vi "读取秘钥.vi"(8 "error in (no error)":errorcluster caption="错误输入（无错误）") -> (0 "error out":errorcluster caption="错误输出", 2 "值":string[](array[string]), 3 "包含启动项":bool)   [LabVIEW 2016]
uses:
  <vilib>/registry/registry.llb/Registry RtKey.ctl
  <vilib>/registry/registry.llb/Read Registry Value Simple STR.vi
panel:
  out "名称":string[](array[string])
  in  "簇":cluster{"password":string}={"password"="平台数据发送系统"}
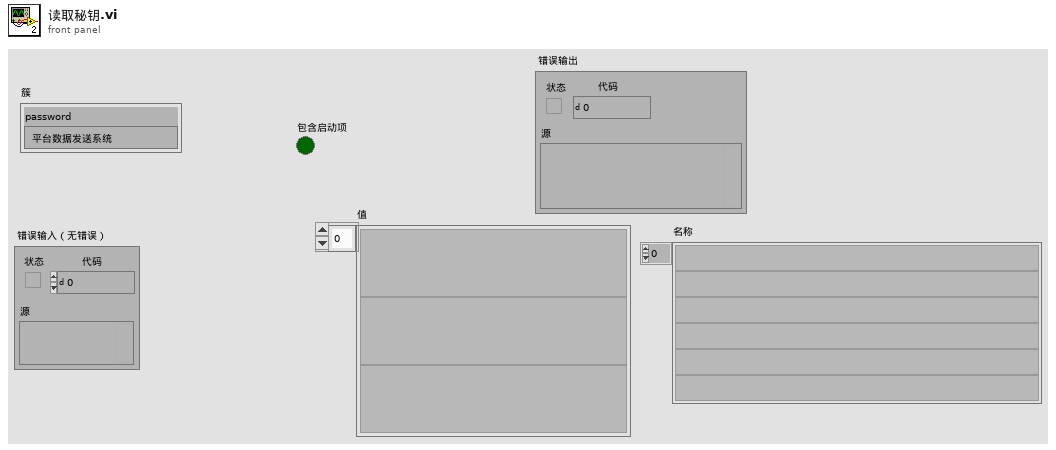
[diagram p1: front panel]
types:
  T1 = typedef "Registry RtKey.ctl" = enum32{"HKEY_CLASSES_ROOT", "HKEY_CURRENT_USER", "HKEY_LOCAL_MACHINE", "HKEY_USERS", "HKEY_PERFORMANCE_DATA", "HKEY_CURRENT_CONFIG", "HKEY_DYN_DATA"}
  T2 = typedef "Registry refnum.ctl" = refnum<k1>
  T3 = cluster{"numValues":i32, "maxValueNameLen":i32, "maxValueDataLen":i32}
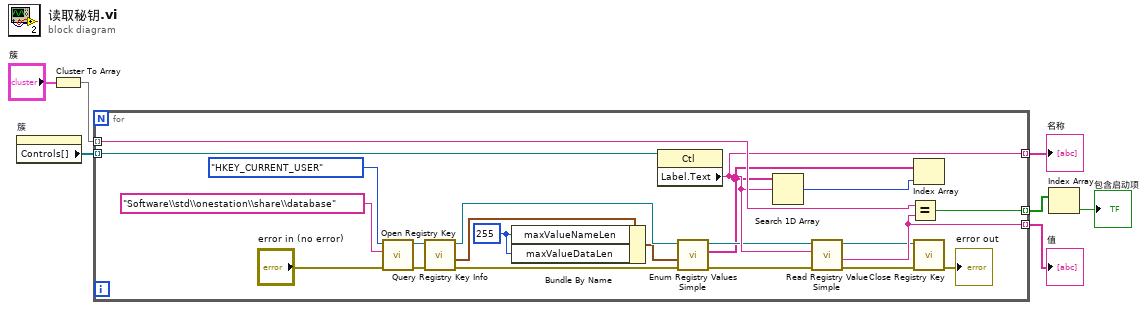
[diagram p0: block diagram]
diagram:
  n1 = property on="簇" class="Clust (严格)"() -> ("Controls[]"=w5:refnum<vi>[])  [unwired: 2 in, 2 out]
  n2 = Cluster To Array(cluster="簇") -> (array=w6:string[])
  n3 = for {
    tunnel: w6 -> [w29] mode=indexing
    tunnel: w5 -> [w28] mode=indexing
    tunnel: [w27] -> w4 mode=indexing
    tunnel: [w26] -> w2 mode=indexing
    tunnel: [w25] -> w3 mode=indexing
    w9 = 255 ("maxValueNameLen")
    n4 = call <vilib>:"Open Registry Key.vi"("error in (no error)"="error in (no error)", "subkey"="Software\\std\\onestation\\share\\database", "root key (HKEY_LOCAL_MACHINE)"=Registry_RtKey."HKEY_CURRENT_USER") -> ("error out"=w21:errorcluster, "refnum out"=w22:T2)  [unwired: 7 in]
    n5 = call <vilib>:"Query Registry Key Info.vi"("error in (no error)"=w21, "refnum"=w22) -> ("error out"=w17:errorcluster, "value info"=w11:T3, "refnum out"=w18:T2)  [unwired: 5 in, 2 out]
    n6 = Bundle By Name(cluster=w11, "maxValueNameLen"=w9, "maxValueDataLen"=w9) -> (w10:T3)
    n7 = property class="Ctl"(reference=w28) -> ("Label.Text"=w25:string)  [unwired: 1 in, 2 out]
    n8 = call <vilib>:"Enum Registry Values Simple.vi"("error in (no error)"=w17, "value info"=w10, "refnum"=w18) -> ("error out"=w14:errorcluster, "values"=w8:string[], "refnum out"=w16:T2)  [unwired: 3 in, 3 out]
    n9 = Search 1D Array(1D array=w8, element=w25) -> (index of element=w12:i32)  [unwired: 1 in]
    n10 = call-poly <vilib>:"Read Registry Value Simple.vi"("error in (no error)"=w14, "value"=w25, "refnum"=w16) -> ("error out"=w13:errorcluster, "String/Binary data"=w27:string, "refnum out"=w15:T2)  [unwired: 3 in, 1 out]
    n11 = Equal?(x=w29, y=w27) -> (x = y?=w26:bool)
    n12 = Index Array(array=w8, index=w12) -> ()  [unwired: 1 out]
    n13 = call <vilib>:"Close Registry Key.vi"("error in (no error)"=w13, "refnum"=w15) -> ("error out"=→"error out":errorcluster)  [unwired: 5 in]
  }
  "值" <- w4
  "名称" <- w3
  n14 = Index Array(array=w2) -> (element=→"包含启动项":bool)  [unwired: 1 in]
